vi "MoveSirah.cm-1.vi"(11 "DyeLaser":T2) -> (3 "output cluster":T1)   [LabVIEW 2022 SP3]
uses:
  Sirah Control API.llb/SC API Unit.ctl
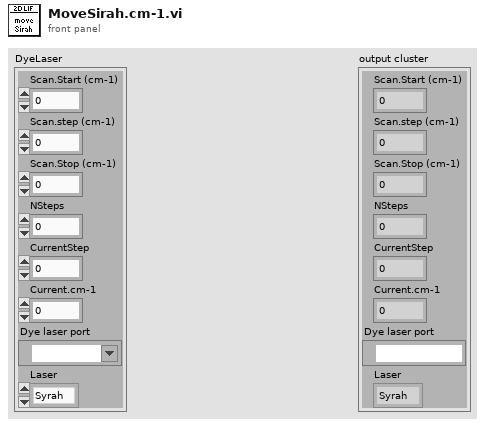
[diagram p1: front panel]
types:
  T1 = cluster{"Scan.Start (cm-1)":dbl, "Scan.Stop (cm-1)":dbl, "Scan.step (cm-1)":dbl, "Dye laser port":refnum<visa-resource-name>, "Laser":enum16{"Syrah", "Hyperdye"}, "NSteps":i32, "CurrentStep":i32, "Current.cm-1":dbl}
  T2 = cluster{"Scan.Start (cm-1)":dbl, "Scan.Stop (cm-1)":dbl, "Scan.step (cm-1)":dbl, "Dye laser port":refnum<visa-resource-name>, "Laser":enum16{"Syrah", "Hyperdye"}, "CurrentStep":i32, "NSteps":i32, "Current.cm-1":dbl}
  T3 = typedef "SC API Unit.ctl" = enum16{"nm", "THz", "1/cm"}
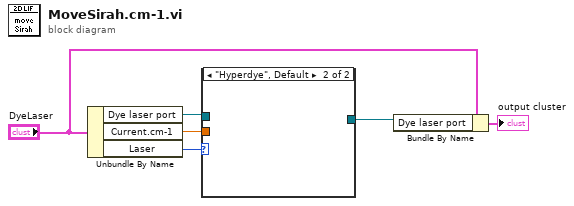
[diagram p0: block diagram]
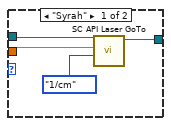
[diagram p2: hidden frame]
diagram:
  n1 = Unbundle By Name("DyeLaser") -> ("Dye laser port"=w5:refnum<visa-resource-name>, "Current.cm-1"=w4:dbl, "Laser"=w6:enum16{"Syrah", "Hyperdye"})
  n2 = case shown="\"Hyperdye\", Default" w6 {
    tunnel: w4 -> [w9 _]
    tunnel: w5 -> [w8 _]
    tunnel: [w7 _] -> w1
    frame "Syrah" {
      n3 = call "SC API Laser GoTo.vi"("Unit"=SC_API_Unit."1/cm", "Wavelength (nm)"=w9, "VISA Resource Name"=w8) -> ("VISA Resource Name Out"=w7:refnum<visa-resource-name>)  [unwired: 7 in, 1 out]
    }
    frame "Hyperdye", Default {
    }
  }
  n4 = Bundle By Name(cluster="DyeLaser", "Dye laser port"=w1) -> (→"output cluster":T2)
